vi "Build FFT Results.vi"(6 "ID/Condition":string[](array[string]), 7 "data info":string[](array[string])=["-1", "-1"], 8 "Freq data":string[][](array[string]), 9 "Write SD":bool=TRUE, 10 "Mean":bool caption="Is Mean", 11 "Panel Refs":T1) -> (3 "FFT Results":string[][](array[string]))   [LabVIEW 2016]
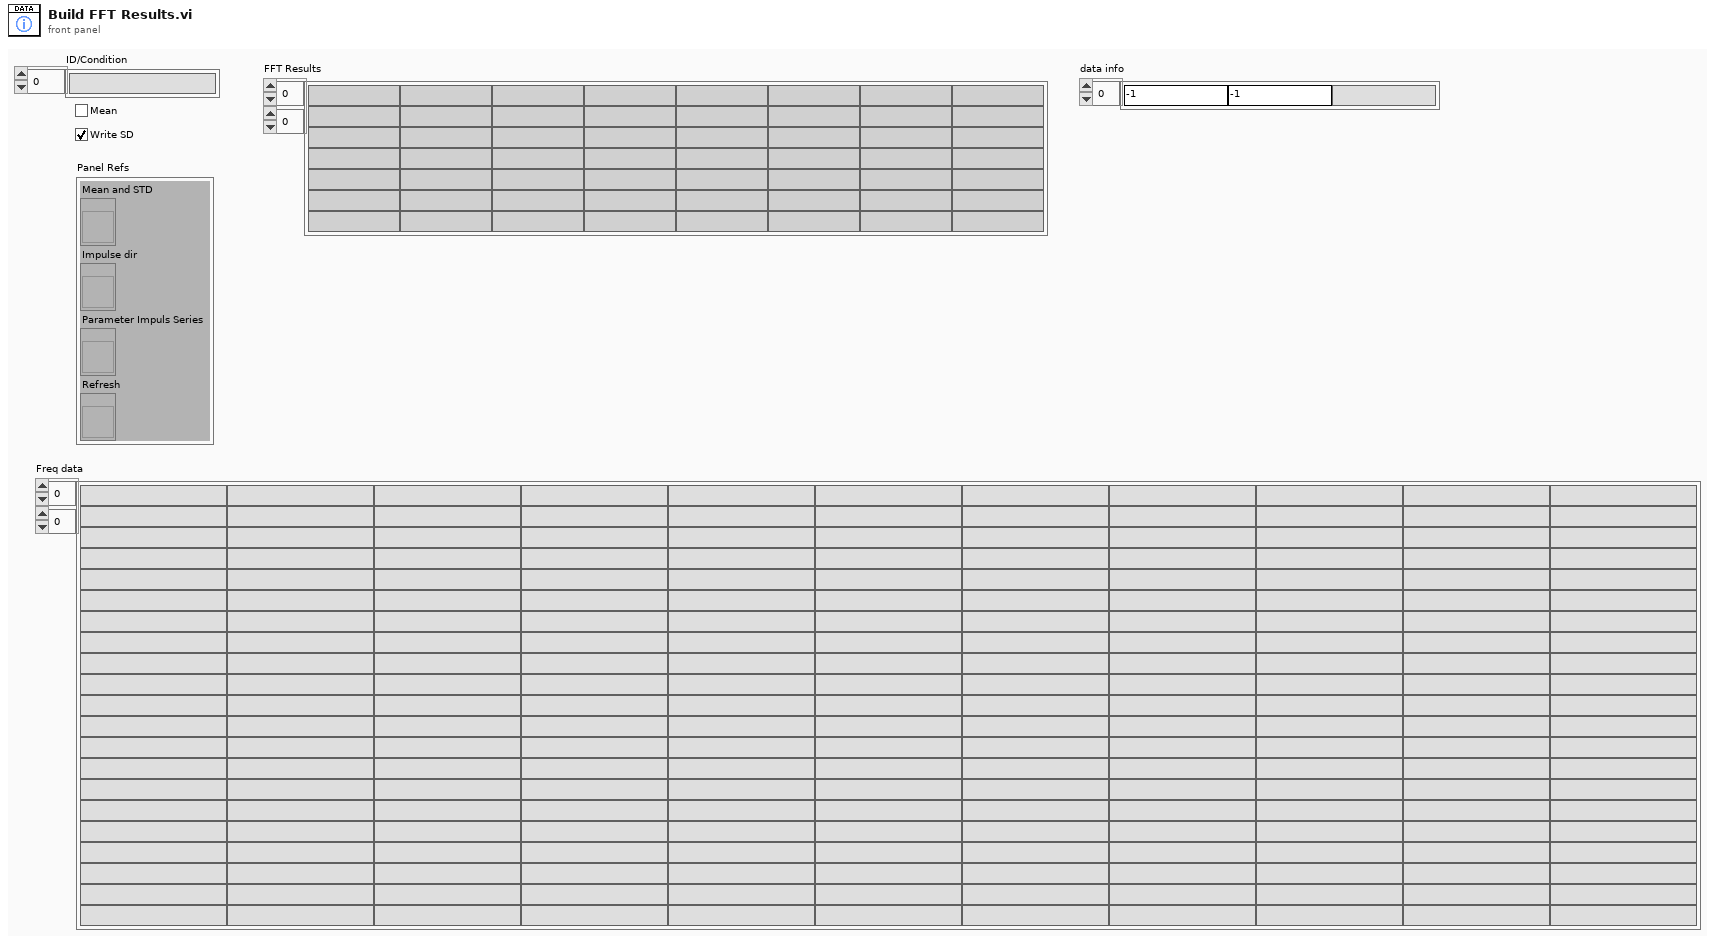
[diagram p1: front panel]
types:
  T1 = cluster{"Mean and STD":refnum<vi>, "Impulse dir":refnum<vi>, "Parameter Impuls Series":refnum<vi>, "Refresh":refnum<vi>}
  T2 = typedef "core.lvlib/TD_Impulse Parameter.ctl" = cluster{"Color":u32, "Visible":bool, "Channel":u16, "Invert":bool, "Desaccade":bool, "Offset":dbl, "Gain":dbl}[]
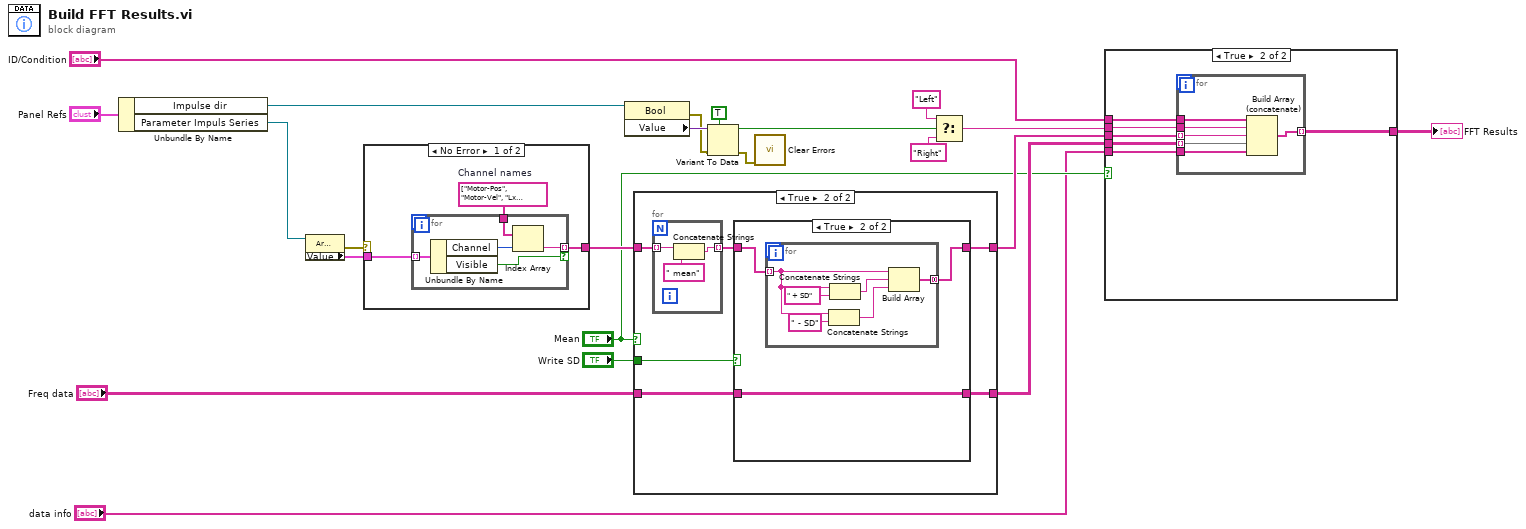
[diagram p0: block diagram]
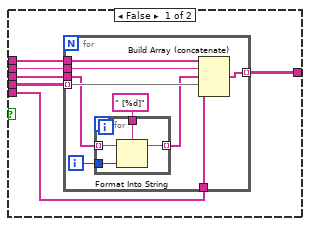
[diagram p2: hidden frame]
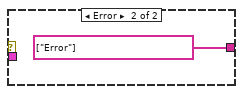
[diagram p3: hidden frame]
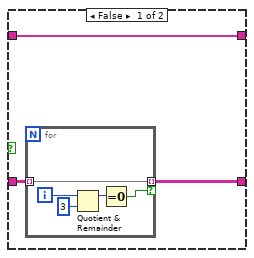
[diagram p5: hidden frame]
diagram:
  n1 = Unbundle By Name("Panel Refs") -> ("Impulse dir"=w22:refnum<vi>, "Parameter Impuls Series"=w13:refnum<vi>)
  n2 = property class="Arr (strict)"(reference=w13) -> (error out=w6:errorcluster, "Value"=w14:T2)  [unwired: 1 in, 1 out]
  n3 = case shown="No Error" w6 {
    tunnel: w14 -> [w25 _]
    tunnel: [w23 string[] ["Error"]] -> w12
    frame No Error {
      w24 = string[] ["Motor-Pos", "Motor-Vel", "Lx Position-in-Head", "Ly Position-in-Head", "Lz Position-in-Head", "Lx Velocity-in-Head", "Ly Velocity-in-Head", "Lz Velocity-in-Head", "Ll Velocity-in-Head", "Lr Velocity-in-Head", "Lx Accel-in-Head", "Ly Accel-in-Head", "Lz Accel-in-Head", "Rx Position-in-Head", "Ry Position-in-Head", "Rz Position-in-Head", "Rx Velocity-in-Head", "Ry Velocity-in-Head", "Rz Velocity-in-Head", "Rl Velocity-in-Head", "Rr Velocity-in-Head", "Rx Accel-in-Head", "Ry Accel-in-Head", "Rz Accel-in-Head", "Global Trigger", "\t", "\t", "\tNA"]  # Channel names
      n4 = for {
        tunnel: w25 -> [w30] mode=indexing
        tunnel: [w26] -> w23 mode=indexing if=w29
        tunnel: w24 -> [w28]
        n5 = Unbundle By Name(w30) -> ("Channel"=w27:u16, "Visible"=w29:bool)
        n6 = Index Array(array=w28, index=w27) -> (element=w26:string)
      }
    }
    frame Error {
    }
  }
  n7 = property class="Bool"(reference=w22) -> (error out=w18:errorcluster, "Value"=w21:variant)  [unwired: 1 in, 1 out]
  n8 = case shown="True" "Mean" {
    tunnel: w12 -> [w33 w39]
    tunnel: [w33 w37] -> w11
    tunnel: "Write SD" -> [_ w36]
    tunnel: "Freq data" -> [w32 w35]
    tunnel: [w32 w34] -> w7
    frame False {
    }
    frame True {
      n9 = for {
        tunnel: w39 -> [w59] mode=indexing
        tunnel: [w57] -> w38 mode=indexing
        n10 = Concatenate Strings(w59, " mean" ("string")) -> (w57:string)
      }
      n11 = case shown="True" w36 {
        tunnel: w38 -> [w42 w50]
        tunnel: [w42 w49] -> w37
        tunnel: w35 -> [w41 w48]
        tunnel: [w40 w48] -> w34
        frame False {
          n12 = for {
            tunnel: w41 -> [w45] mode=indexing
            tunnel: [w45] -> w40 mode=indexing if=w43
            i -> [w47]
            n13 = Quotient & Remainder(x=w47, y=3) -> (x-y*floor(x/y)=w44:i32)  [unwired: 1 out]
            n14 = Equal To 0?(x=w44) -> (x = 0?=w43:bool)
          }
        }
        frame True {
          n15 = for {
            tunnel: w50 -> [w54] mode=indexing
            tunnel: [w51] -> w49 mode=concatenating
            n16 = Concatenate Strings(w54, " - SD" ("string")) -> (w52:string)
            n17 = Concatenate Strings(w54, " + SD" ("string")) -> (w53:string)
            n18 = Build Array(w54, w53, w52) -> (w51:string[])
          }
        }
      }
    }
  }
  n19 = Variant To Data(error in=w18, type=TRUE, Variant=w21) -> (data=w19:bool, error out=w5:errorcluster)
  n20 = call <vilib>:"Clear Errors.vi"("error in (no error)"=w5) -> ()  [unwired: 5 in, 2 out]
  n21 = Select(t="Left", s=w19, f="Right") -> (s? t:f=w15:string)
  n22 = case shown="True" "Mean" {
    tunnel: w15 -> [w65 w84]
    tunnel: w11 -> [w64 w83]
    tunnel: "ID/Condition" -> [w63 w82]
    tunnel: w7 -> [w62 w81]
    tunnel: [w61 w80] -> w4
    tunnel: "data info" -> [w60 w79]
    frame False {
      n23 = for {
        tunnel: w65 -> [w74]
        tunnel: w64 -> [w69]
        tunnel: w63 -> [w73]
        tunnel: w62 -> [w71] mode=indexing
        tunnel: [w67] -> w61 mode=indexing
        tunnel: w60 -> [w66]
        i -> [w70]
        n24 = for {
          tunnel: w70 -> [w78]
          tunnel: [w77] -> w68 mode=indexing
          tunnel: w69 -> [w76] mode=indexing
          tunnel: " [%d]" ("format string") -> [w75]
          n25 = Format Into String(format string=w75, initial string=w76, w78) -> (resulting string=w77:string)  [unwired: 1 in, 1 out]
        }
        n26 = Build Array (concatenate)(w73, w74, w68, w71, w66) -> (w67:string[])
      }
    }
    frame True {
      n27 = for {
        tunnel: w84 -> [w90]
        tunnel: w83 -> [w86] mode=indexing
        tunnel: w82 -> [w89]
        tunnel: w81 -> [w88] mode=indexing
        tunnel: [w87] -> w80 mode=indexing
        tunnel: w79 -> [w85]
        n28 = Build Array (concatenate)(w89, w90, w86, w88, w85) -> (w87:string[])
      }
    }
  }
  "FFT Results" <- w4
